vi "Daq.Simulator.vi"() -> ()   [LabVIEW 2016]
uses:
  Drivers/FestoCPX/FestoCPX.DO.Data.Fglb.Action.ctl
  Drivers/FestoCPX/FestoCPX.DI.Data.Fglb.Action.ctl
  Global/ApplicationGlobal.vi
  Drivers/FestoCPX/FestoCPX.Global.vi
panel:
  out "DO":i32(listbox) caption="DO CPX"
  in  "DI.Butt":bool[](array[boolean])=[TRUE, TRUE, TRUE, TRUE, TRUE, TRUE, FALSE, FALSE, FALSE, TRUE, TRUE, FALSE, FALSE, TRUE, TRUE, TRUE, TRUE, FALSE, TRUE, FALSE, FALSE, FALSE, FALSE, FALSE, FALSE, FALSE, FALSE, FALSE, FALSE, FALSE, FALSE, FALSE, FALSE, FALSE, FALSE, TRUE, TRUE, TRUE, TRUE]
  out "DI":i32(listbox) caption="DI CPX"
  out "Panel":refnum<vi>
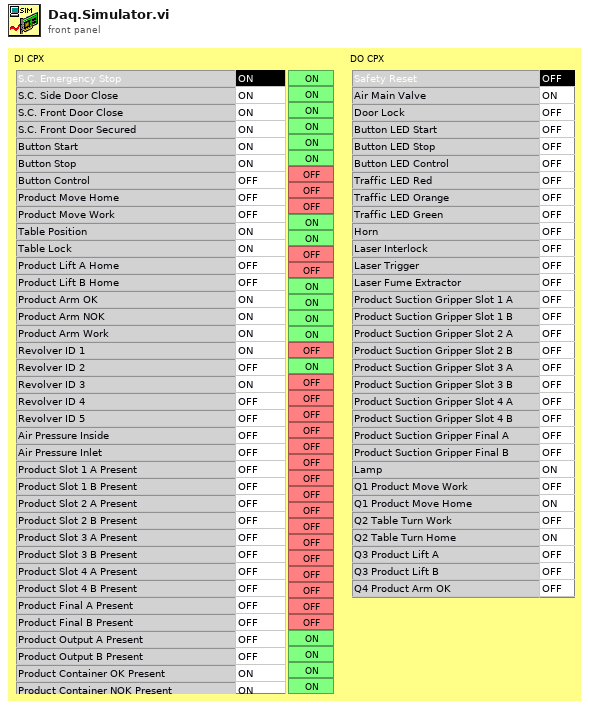
[diagram p1: front panel]
types:
  T1 = enum32{"Invalid", "Standard", "Closed", "Hidden", "Minimized", "Maximized"}
  T2 = typedef "FestoCPX.DO.Data.Fglb.Action.ctl" = enum16{"init", "set", "get", "check", "select", "reset"}
  T3 = typedef "FestoCPX.DI.Data.Fglb.Action.ctl" = enum16{"init", "set", "simul", "get"}
  T4 = typedef "FestoCPX.Data.Sets.ctl" = cluster{"IP":string, "Timeout_ms":i32, "ReconnectPeriod_s":i32, "Config.DI":T5[], "Config.DO":T7[]}
  T5 = typedef "FestoCPX.DI.Sets.ctl" = cluster{"Name":string, "Channel":T6, "Negate":bool}
  T6 = typedef "FestoCPX.DI.ctl" = enum16{"0.0", "0.1", "0.2", "0.3", "0.4", "0.5", "0.6", "0.7", "1.0", "1.1", "1.2", "1.3", "1.4", "1.5", "1.6", "1.7", "2.0", "2.1", "2.2", "2.3", "2.4", "2.5", "2.6", "2.7", "3.0", "3.1", "3.2", "3.3", "3.4", "3.5", "3.6", "3.7", "4.0", "4.1", "4.2", "4.3", "4.4", "4.5", "4.6", "4.7"}
  T7 = typedef "FestoCPX.DO.Sets.ctl" = cluster{"Name":string, "Channel":T8, "Negate":bool, "Default":bool}
  T8 = typedef "FestoCPX.DO.ctl" = enum16{"4.0", "4.1", "4.2", "4.3", "4.4", "4.5", "4.6", "4.7", "5.0", "5.1", "5.2", "5.3", "5.4", "5.5", "5.6", "5.7", "6.0", "6.1", "6.2", "6.3", "6.4", "6.5", "6.6", "6.7", "Q1K1", "Q1K2", "Q2K1", "Q2K2", "Q3K1", "Q3K2", "Q4K1", "Q4K2", "Q5K1", "Q5K2", "Q6K1", "Q6K2"}
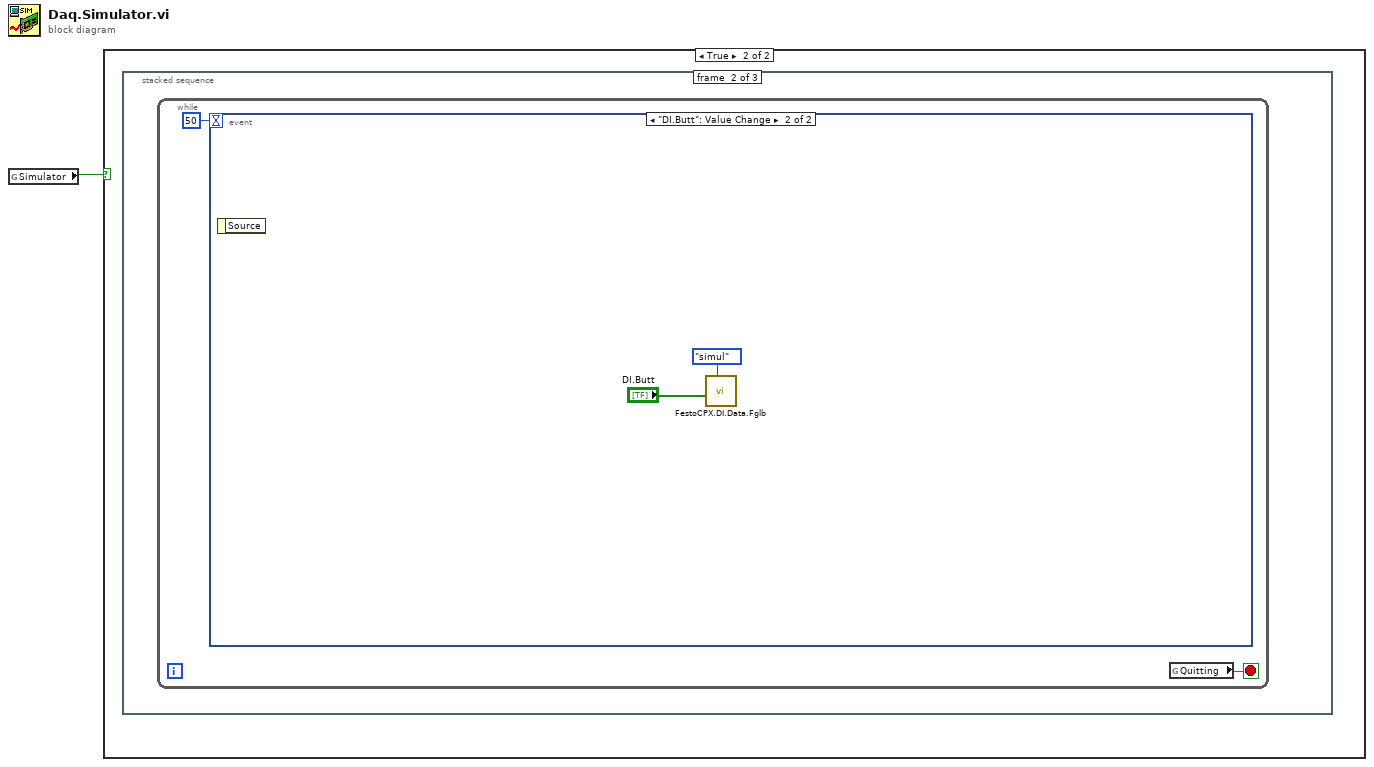
[diagram p0: block diagram]
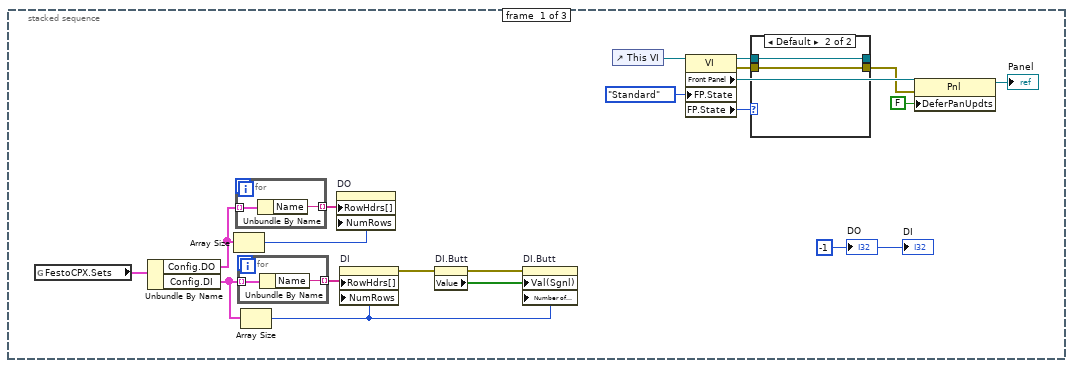
[diagram p3: hidden frame]
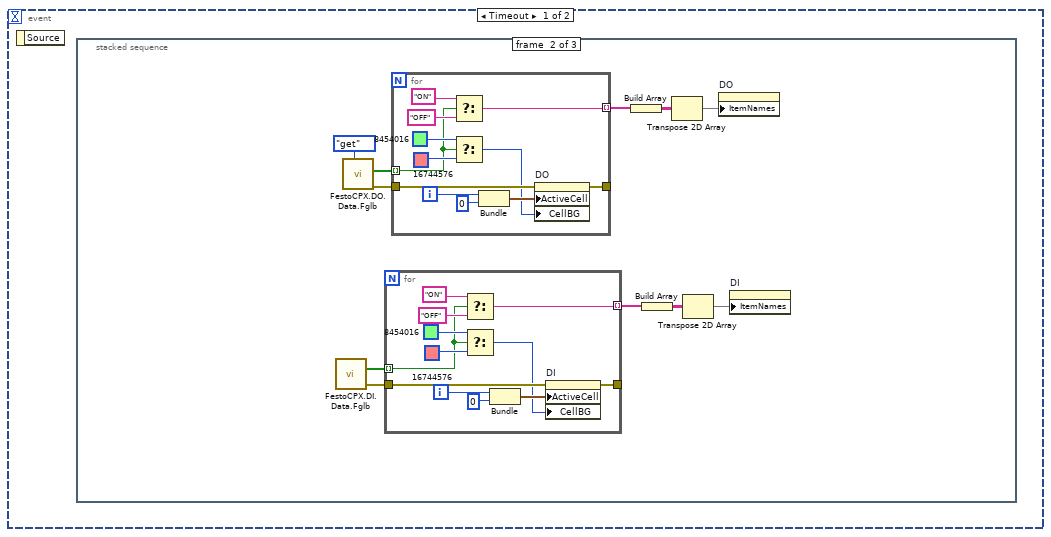
[diagram p5: hidden frame]
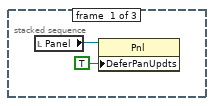
[diagram p6: hidden frame]
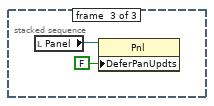
[diagram p7: hidden frame]
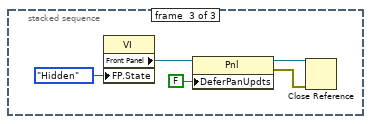
[diagram p8: hidden frame]
diagram:
  n1 = global read "ApplicationGlobal.vi" "Simulator"() -> (w1:bool)
  n2 = case shown="True" w1 {
    frame False {
    }
    frame True {
      n3 = stacked-sequence {
        frame #0 {
          w3 = -1 ("Daq.DO")
          n4 = global read "FestoCPX.Global.vi" "FestoCPX.Sets"() -> (w4:T4)
          n5 = Unbundle By Name(w4) -> ("Config.DO"=w9:T7[], "Config.DI"=w8:T5[])
          n6 = Array Size(array=w9) -> (size(s)=w7:i32)
          n7 = for {
            tunnel: w9 -> [w23] mode=indexing
            tunnel: [w22] -> w5 mode=indexing
            n8 = Unbundle By Name(w23) -> ("Name"=w22:string)
          }
          n9 = for {
            tunnel: w8 -> [w25] mode=indexing
            tunnel: [w24] -> w6 mode=indexing
            n10 = Unbundle By Name(w25) -> ("Name"=w24:string)
          }
          n11 = Array Size(array=w8) -> (size(s)=w10:i32)
          n12 = property on="DO" class="MCListbox (strict)"("RowHdrs[]"=w5, "NumRows"=w7) -> ()  [unwired: 2 in, 2 out]
          n13 = property on="DI" class="MCListbox (strict)"("RowHdrs[]"=w6, "NumRows"=w10) -> (error out=w12:errorcluster)  [unwired: 2 in, 1 out]
          n14 = property on="DI.Butt" class="Arr (strict)"(error in=w12) -> (error out=w13:errorcluster, "Value"=w11:bool[])  [unwired: 1 in, 1 out]
          n15 = property on="DI.Butt" class="Arr (strict)"(error in=w13, "Val(Sgnl)"=w11, "Number of Rows"=w10) -> ()  [unwired: 1 in, 2 out]
          n16 = control-ref of="This VI"() -> (w19:refnum<vi>)
          n17 = property class="VI"(reference=w19, "FP.State"=T1."Standard" ("Front Panel Window:State")) -> (reference out=w18:refnum<vi>, error out=w17:errorcluster, "Front Panel"=w21:refnum<vi>, "FP.State"=w15:T1)  [unwired: 1 in]
          n18 = case shown="Default" w15 {
            tunnel: w18 -> [w27 w29]
            tunnel: w17 -> [w26 w28]
            tunnel: [w27 w29] -> _
            tunnel: [w26 w28] -> w16
            frame "Invalid", "Closed" {
            }
            frame Default {
            }
          }
          n19 = property class="Pnl"(reference=w21, error in=w16, "DeferPanUpdts"=FALSE ("Defer Panel Updates")) -> (reference out=→"Panel":refnum<vi>)  [unwired: 1 out]
          "DO" <- w3
          "DI" <- w3
        }
        frame #1 {
          n20 = while {
            stop <- w31 stop-if-true
            n21 = event shown="[1] \"DI.Butt\": Value Change" {
              selector: _ -> [_ _]
              dyn-events: _ -> [_ _]
              timeout: 50 -> [_ _]
              event Timeout {
                n22 = event-data() -> ()  [unwired: 1 in, 1 out]
                n23 = stacked-sequence {
                  frame #0 {
                    n24 = local read "Panel"() -> (w33:refnum<vi>)
                    n25 = property class="Pnl"(reference=w33, "DeferPanUpdts"=TRUE ("Defer Panel Updates")) -> ()  [unwired: 1 in, 2 out]
                  }
                  frame #1 {
                    n26 = call "FestoCPX.DI.Data.Fglb.vi"() -> ("error out"=w36:errorcluster, "data out"=w34:bool[])  [unwired: 7 in, 3 out]
                    n27 = call "FestoCPX.DO.Data.Fglb.vi"("state (get all)"=FestoCPX.DO.Data.Fglb.Action."get") -> ("error out"=w41:errorcluster, "State out"=w42:bool[])  [unwired: 8 in, 1 out]
                    n28 = for {
                      tunnel: [w51] -> w39 mode=indexing
                      tunnel: w36 -> [w56]
                      tunnel: [w55] -> _
                      tunnel: w34 -> [w45] mode=indexing
                      i -> [w50]
                      n29 = Select(t="ON" ("string"), s=w45, f="OFF" ("string")) -> (s? t:f=w51:string)
                      n30 = Select(t=u32 8454016, s=w45, f=u32 16744576) -> (s? t:f=w52:u32)
                      n31 = Bundle(w50, 0) -> (w53:cluster{i32, i32})  [unwired: 1 in]
                      n32 = property on="DI" class="MCListbox (strict)"(error in=w56, "ActiveCell"=w53, "CellBG"=w52) -> (error out=w55:errorcluster)  [unwired: 1 in, 1 out]
                    }
                    n33 = for {
                      tunnel: [w63] -> w40 mode=indexing
                      tunnel: w41 -> [w68]
                      tunnel: [w67] -> _
                      tunnel: w42 -> [w57] mode=indexing
                      i -> [w62]
                      n34 = Select(t="ON" ("string"), s=w57, f="OFF" ("string")) -> (s? t:f=w63:string)
                      n35 = Select(t=u32 8454016, s=w57, f=u32 16744576) -> (s? t:f=w64:u32)
                      n36 = Bundle(w62, 0) -> (w65:cluster{i32, i32})  [unwired: 1 in]
                      n37 = property on="DO" class="MCListbox (strict)"(error in=w68, "ActiveCell"=w65, "CellBG"=w64) -> (error out=w67:errorcluster)  [unwired: 1 in, 1 out]
                    }
                    n38 = Build Array(w40) -> (w43:string[][])
                    n39 = Build Array(w39) -> (w38:string[][])
                    n40 = Transpose 2D Array(2D array=w43) -> (transposed array=w44:string[][])
                    n41 = Transpose 2D Array(2D array=w38) -> (transposed array=w37:string[][])
                    n42 = property on="DO" class="MCListbox (strict)"("ItemNames"=w44) -> ()  [unwired: 2 in, 2 out]
                    n43 = property on="DI" class="MCListbox (strict)"("ItemNames"=w37) -> ()  [unwired: 2 in, 2 out]
                  }
                  frame #2 {
                    n44 = local read "Panel"() -> (w70:refnum<vi>)
                    n45 = property class="Pnl"(reference=w70, "DeferPanUpdts"=FALSE ("Defer Panel Updates")) -> ()  [unwired: 1 in, 2 out]
                  }
                }
              }
              event "DI.Butt": Value Change {
                n46 = event-data() -> ()  [unwired: 1 in, 1 out]
                n47 = call "FestoCPX.DI.Data.Fglb.vi"("state (get)"=FestoCPX.DI.Data.Fglb.Action."simul", "data bool"="DI.Butt") -> ()  [unwired: 5 in, 5 out]
              }
            }
            n48 = global read "ApplicationGlobal.vi" "Quitting"() -> (w31:bool)
          }
        }
        frame #2 {
          n49 = property class="VI"("FP.State"=T1."Hidden" ("Front Panel Window:State")) -> ("Front Panel"=w73:refnum<vi>)  [unwired: 2 in, 2 out]
          n50 = property class="Pnl"(reference=w73, "DeferPanUpdts"=FALSE ("Defer Panel Updates")) -> (reference out=w76:refnum<vi>, error out=w75:errorcluster)  [unwired: 1 in]
          n51 = Close Reference(reference=w76, error in (no error)=w75) -> ()  [unwired: 1 out]
        }
      }
    }
  }
